vi "AnalysisGUI.Initialize.vi"(8 "error in (no error)":errorcluster, 9 "DUTs":string[](array[string]), 10 "Use?":bool[](array[boolean]), 11 "Refs":T1) -> (0 "error out":errorcluster, 2 "Tree Strings":string[](array[string]), 3 "Refs":T1)   [LabVIEW 2014, in "NIAnalysis.lvlib"]
uses:
  NIAnalysis.lvlib
  Types/AnalysisGUI.Refs.ctl
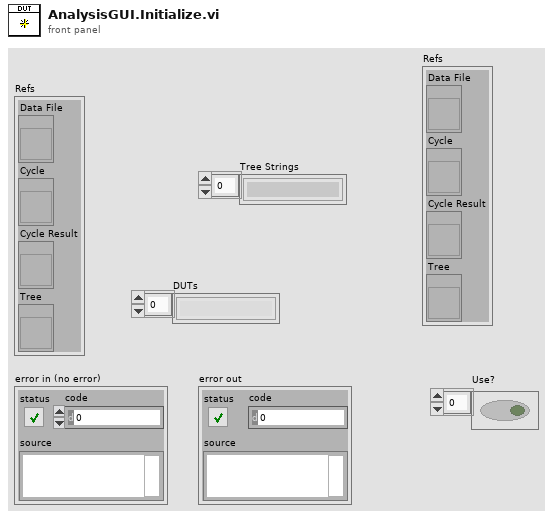
[diagram p1: front panel]
types:
  T1 = typedef "NIAnalysis.lvlib/AnalysisGUI.Refs.ctl" = cluster{"Data File":refnum<vi>, "Cycle":refnum<vi>, "Cycle Result":refnum<vi>, "Tree":refnum<vi>}
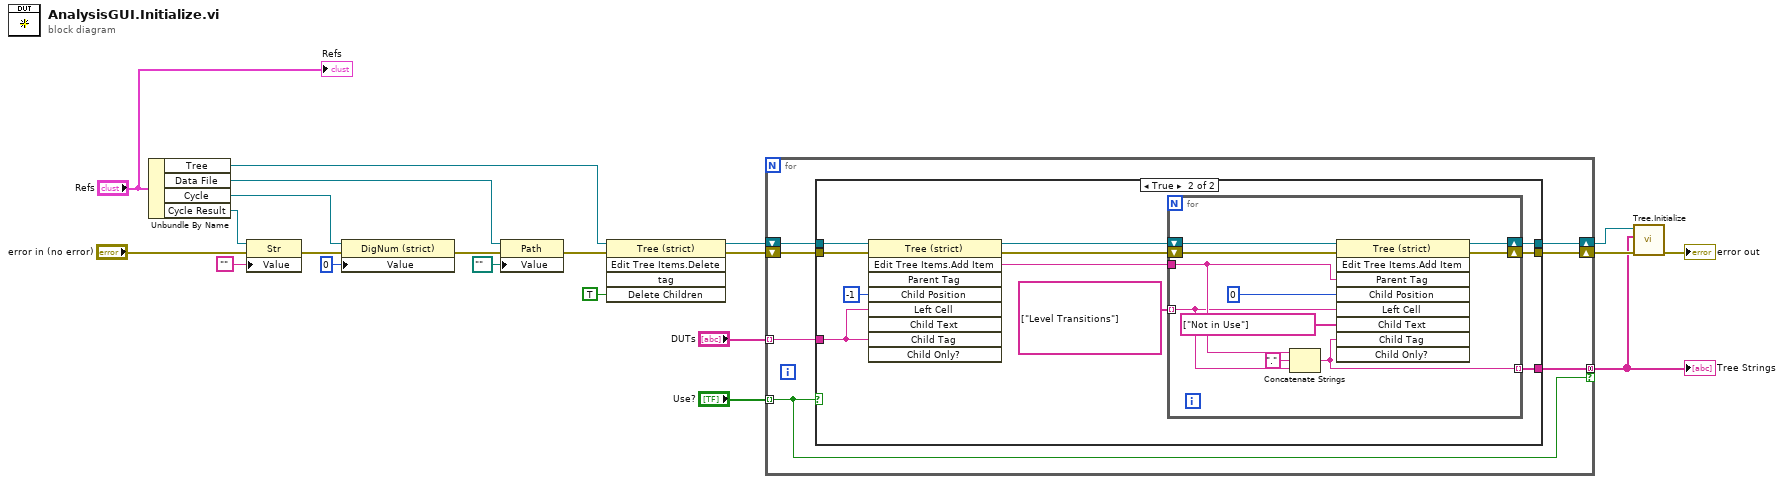
[diagram p0: block diagram]
diagram:
  n1 = Unbundle By Name("Refs") -> ("Tree"=w21:refnum<vi>, "Data File"=w10:refnum<vi>, "Cycle"=w11:refnum<vi>, "Cycle Result"=w14:refnum<vi>)
  n2 = property class="Str"(reference=w14, error in="error in (no error)", "Value"="") -> (error out=w9:errorcluster)  [unwired: 1 out]
  n3 = property class="DigNum (strict)"(reference=w11, error in=w9, "Value"=0) -> (error out=w7:errorcluster)  [unwired: 1 out]
  n4 = property class="Path"(reference=w10, error in=w7, "Value"=path "") -> (error out=w5:errorcluster)  [unwired: 1 out]
  n5 = invoke class="Tree (strict)" method="Edit Tree Items.Delete"(reference=w21, error in=w5, "Delete Children"=TRUE ("Delete Children?")) -> (reference out=w16:refnum<vi>, error out=w17:errorcluster)  [unwired: 2 in, 3 out]
  n6 = for {
    shift-right: [w27] -> w19
    shift-left: w16 -> [w28]
    tunnel: [w24] -> w2 mode=concatenating if=w23
    shift-right: [w25] -> w18
    shift-left: w17 -> [w26]
    tunnel: "Use?" -> [w23] mode=indexing
    tunnel: "DUTs" -> [w22] mode=indexing
    n7 = case shown="True" w23 {
      tunnel: w28 -> [w30 w41]
      tunnel: [w30 w40] -> w27
      tunnel: w26 -> [w29 w39]
      tunnel: [w29 w38] -> w25
      tunnel: [_ w32] -> w24
      tunnel: w22 -> [_ w31]
      frame False {
      }
      frame True {
        n8 = invoke class="Tree (strict)" method="Edit Tree Items.Add Item"(reference=w41, error in=w39, "Child Position"=-1, "Left Cell"=w31, "Child Tag"=w31) -> (reference out=w37:refnum<vi>, error out=w36:errorcluster, "Edit Tree Items:Add Item"=w35:string)  [unwired: 4 in, 6 out]
        n9 = for {
          tunnel: w35 -> [w47]
          tunnel: string[] ["Level Transitions"] -> [w45] mode=indexing
          shift-right: [w44] -> w40
          shift-left: w37 -> [w51]
          tunnel: [w43] -> w32 mode=indexing
          shift-right: [w42] -> w38
          shift-left: w36 -> [w50]
          n10 = Concatenate Strings(w47, "." ("string"), w45) -> (w43:string)
          n11 = invoke class="Tree (strict)" method="Edit Tree Items.Add Item"(reference=w51, error in=w50, "Parent Tag"=w47, "Child Position"=0, "Left Cell"=w45, "Child Text"=string[] ["Not in Use"], "Child Tag"=w43) -> (reference out=w44:refnum<vi>, error out=w42:errorcluster)  [unwired: 2 in, 7 out]
        }
      }
    }
  }
  "Tree Strings" <- w2
  n12 = call "Tree.Initialize.vi"("error in (no error)"=w18, "Tree Strings"=w2, "TreeControl"=w19) -> ("error out"=→"error out":errorcluster)  [unwired: 7 in, 1 out]
  "Refs" <- "Refs"
